vi "Test program 4.vi"() -> ()   [LabVIEW 2013, in "Keithly user program.lvlib"]
uses:
  Keithly user program.lvlib
  Typedefs/KE622x -- On Off Control.ctl
  Configure/Output/Typedefs/KE6221 -- Output Response.ctl
  Configure/Source/Typedefs/KE622x -- Current Range.ctl
  Configure/Source/Typedefs/KE622x -- Current Level.ctl
  Configure/Source/Typedefs/KE622x -- Voltage Limit.ctl
  Configure/Utility/Typedefs/KE622x -- Instrument Type.ctl
panel:
  out "XY Graph":cluster{"X":dbl, "Y":dbl}[](graph)
  in  "stop":bool
  in  "2182 -A Params In":T1={"Auto Range?"=FALSE, "Man / Selected\n       Range"=enum."10mV", "Enable Digital\n       Filter?"=FALSE, "Filter Type"=enum."Movin", "Filter Count"=1, "      Filter\nWindow (%)"=0.01, "Enable Analog\n       Filter?"=FALSE, "NPLCs"=5} {"NPLCs" min=1 max=10; "Filter\nWindow (%)" min=0.01 max=10.0 step=0.01 format="%.2f"; "Filter Count" min=1 max=100}
  out "Compliance?":bool
  out "Interlock Tripped?":bool
  in  "Voltage Limit (V)":T2=10.0 min=0.1 max=105.0 step=0.01 format="%.2p"
  in  "Current Level (A)":T3=0.1 min=-0.105 max=0.105 format="%.4p"
  in  "Current Range":T4
  in  "KE6221 Output Response":T5=enum."Slow"
  in  "Analog Filter State":T6
  in  "Check For SCPI Errors? (T)":bool=TRUE
  in  "VISA resource name":refnum<visa-resource-name>
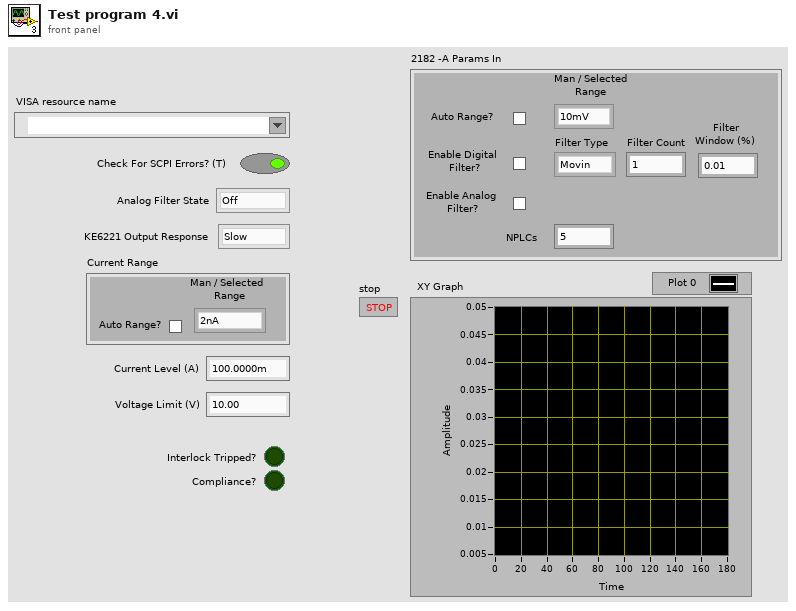
[diagram p1: front panel]
types:
  T1 = cluster{"Auto Range?":bool, "Man / Selected\n       Range":enum16{"10mV", "100mV", "1V", "10V", "100V"}, "Enable Digital\n       Filter?":bool, "Filter Type":enum16{"Movin", "Repeat"}, "Filter Count":u32, "      Filter\nWindow (%)":dbl, "Enable Analog\n       Filter?":bool, "NPLCs":u32}
  T2 = typedef "Keithly user program.lvlib/KE622x -- Voltage Limit.ctl" = dbl
  T3 = typedef "Keithly user program.lvlib/KE622x -- Current Level.ctl" = dbl
  T4 = typedef "Keithly user program.lvlib/KE622x -- Current Range.ctl" = cluster{"Auto Range?":bool, "Man / Selected\n        Range":enum16{"2nA", "20nA", "200nA", "2uA", "20uA", "200uA", "2mA", "20mA", "100mA"}}
  T5 = typedef "Keithly user program.lvlib/KE6221 -- Output Response.ctl" = enum16{"Fast", "Slow"}
  T6 = typedef "Keithly user program.lvlib/KE622x -- On Off Control.ctl" = enum16{"Off", "On"}
  T7 = typedef "Keithly user program.lvlib/KE622x -- Instrument Type.ctl" = enum16{"KE6220", "KE6221"}
  T8 = cluster{"Auto Range?":bool, "Man / Selected\n        Range":u16, "Enable Digital\n       Filter?":bool, "Filter Type":u16, "Filter Count":u32, "      Filter\nWindow (%)":dbl, "Enable Analog\n       Filter?":bool, "NPLCs":u32}
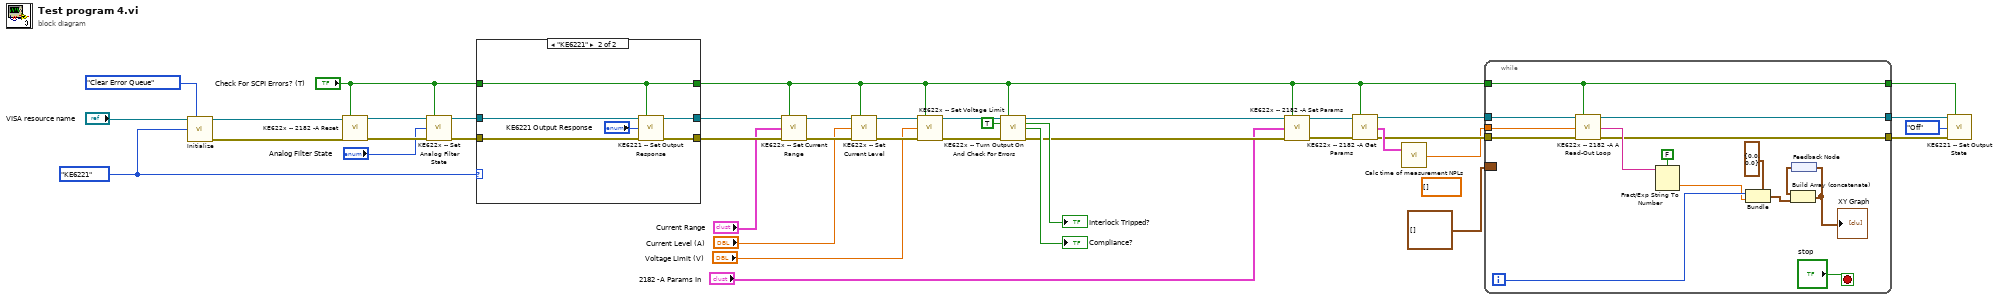
[diagram p0: block diagram]
diagram:
  (unwired) dbl[] []
  w33 = KE622x_--_Instrument_Type."KE6221" ("Instrument Type")
  n1 = call "Initialize.vi"("VISA resource name"="VISA resource name", "Error Queue Option"=enum16{"Clear Error Queue", "Error Query"}."Clear Error Queue", "Instrument Type"=w33) -> ("VISA resource name out"=w39:refnum<visa-resource-name>, "error out"=w38:errorcluster)  [unwired: 11 in]
  n2 = call "KE622x -- 2182 -A Reset.vi"("622x Resource In"=w39, "Check For SCPI Errors? (T)"="Check For SCPI Errors? (T)", "error in (no error)"=w38) -> ("622x Resource Out (dupl)"=w36:refnum<visa-resource-name>, "error out"=w35:errorcluster)  [unwired: 11 in]
  n3 = call "KE622x -- Set Analog Filter State.vi"("Resource In"=w36, "Check For SCPI Errors? (T)"="Check For SCPI Errors? (T)", "Analog Filter State"="Analog Filter State", "error in (no error)"=w35) -> ("Resource Out (dupl)"=w32:refnum<visa-resource-name>, "error out"=w31:errorcluster)  [unwired: 10 in]
  n4 = case shown="\"KE6221\"" w33 {
    tunnel: w32 -> [w42 w49]
    tunnel: w31 -> [w41 w48]
    tunnel: [w43 w44] -> w3
    tunnel: "Check For SCPI Errors? (T)" -> [w43 w44]
    tunnel: [w42 w46] -> w29
    tunnel: [w41 w45] -> w28
    frame "KE6220", Default {
    }
    frame "KE6221" {
      n5 = call "KE6221 -- Set Output Response.vi"("Resource In"=w49, "Check For SCPI Errors? (T)"=w44, "KE6221 Output Response"="KE6221 Output Response", "error in (no error)"=w48) -> ("Resource Out (dupl)"=w46:refnum<visa-resource-name>, "error out"=w45:errorcluster)  [unwired: 10 in]
    }
  }
  n6 = call "KE622x -- Set Current Range.vi"("Resource In"=w29, "Check For SCPI Errors? (T)"=w3, "Current Range"="Current Range", "error in (no error)"=w28) -> ("Resource Out (dupl)"=w26:refnum<visa-resource-name>, "error out"=w25:errorcluster)  [unwired: 10 in]
  n7 = call "KE622x -- Set Current Level.vi"("Resource In"=w26, "Check For SCPI Errors? (T)"=w3, "Current Level (A)"="Current Level (A)", "error in (no error)"=w25) -> ("Resource Out (dupl)"=w23:refnum<visa-resource-name>, "error out"=w22:errorcluster)  [unwired: 10 in]
  n8 = call "KE622x -- Set Voltage Limit.vi"("Resource In"=w23, "Check For SCPI Errors? (T)"=w3, "Voltage Limit (V)"="Voltage Limit (V)", "error in (no error)"=w22) -> ("Resource Out (dupl)"=w20:refnum<visa-resource-name>, "error out"=w19:errorcluster)  [unwired: 10 in]
  n9 = call "KE622x -- Turn Output On And Check For Errors.vi"("Resource In"=w20, "Check For SCPI Errors? (T)"=w3, "Turn Off Output If Compliance?"=TRUE, "error in (no error)"=w19) -> ("Resource Out (dupl)"=w14:refnum<visa-resource-name>, "Interlock Tripped?"=→"Interlock Tripped?":bool, "Compliance?"=→"Compliance?":bool, "error out"=w15:errorcluster)  [unwired: 8 in]
  n10 = call "KE622x -- 2182 -A Set Params.vi"("622x Resource In"=w14, "Check For SCPI Errors? (T)"=w3, "2182 -A Params In"="2182 -A Params In", "error in (no error)"=w15) -> ("622x Resource Out (dupl)"=w13:refnum<visa-resource-name>, "error out"=w12:errorcluster)  [unwired: 10 in]
  n11 = call "KE622x -- 2182 -A Get Params.vi"("622x Resource In"=w13, "Check For SCPI Errors? (T)"=w3, "error in (no error)"=w12) -> ("622x Resource Out (dupl)"=w9:refnum<visa-resource-name>, "2182 -A Params"=w10:T8, "error out"=w8:errorcluster)  [unwired: 10 in]
  n12 = call "Calc time of measurement NPLs.vi"("2182 -A Params"=w10) -> ("Time of one measurement"=w7:dbl)  [unwired: 1 in]
  n13 = while {
    tunnel: w9 -> [w64]
    tunnel: w8 -> [w63]
    tunnel: w7 -> [w62]
    border: cluster{"X":dbl, "Y":dbl}[] [] ("XY Graph") -> [_]
    tunnel: [w58] -> w6
    tunnel: [w57] -> w5
    tunnel: w3 -> [w56]
    tunnel: [w56] -> w2
    i -> [w52]
    stop <- "stop" stop-if-true
    n14 = call "KE622x -- 2182 -A A Read-Out Loop.vi"("622x Resource In"=w64, "Check For SCPI Errors? (T)"=w56, "Time of one measurement"=w62, "error in (no error)"=w63) -> ("622x Resource Out (dupl)"=w58:refnum<visa-resource-name>, "2182-A Reponse String"=w61:string, "error out"=w57:errorcluster)  [unwired: 9 in]
    n15 = Fract/Exp String To Number(use system decimal point (T)=FALSE, string=w61) -> (number=w51:dbl)  [unwired: 2 in, 1 out]
    n16 = Bundle(cluster=cluster{"X":dbl, "Y":dbl} {"X"=0.0, "Y"=0.0}, "X"=w52, "Y"=w51) -> (w53:cluster{"X":dbl, "Y":dbl})
    n17 = feedback #1() -> (w54:cluster{"X":dbl, "Y":dbl}[])
    n18 = Build Array (concatenate)(w54, w53) -> (w50:cluster{"X":dbl, "Y":dbl}[])
    "XY Graph" <- w50
    n19 = feedback-in #1(w50) -> ()
  }
  n20 = call "KE6221 -- Set Output State.vi"("Resource In"=w6, "Check For SCPI Errors? (T)"=w2, "Output State"=KE622x_--_On_Off_Control."Off", "error in (no error)"=w5) -> ()  [unwired: 10 in, 2 out]
